vi "InitGantner.vi"(8 "error in":errorcluster, 10 "Port":i32) -> (0 "error out":errorcluster caption="error in", 2 "Module":T1)   [LabVIEW 2012]
uses:
  Gantner-Instruments ISMBUS32.llb/ISMBUS_Module.ctl
  Gantner-Instruments ISMBUS32.llb/ISMBUS_Channel.ctl
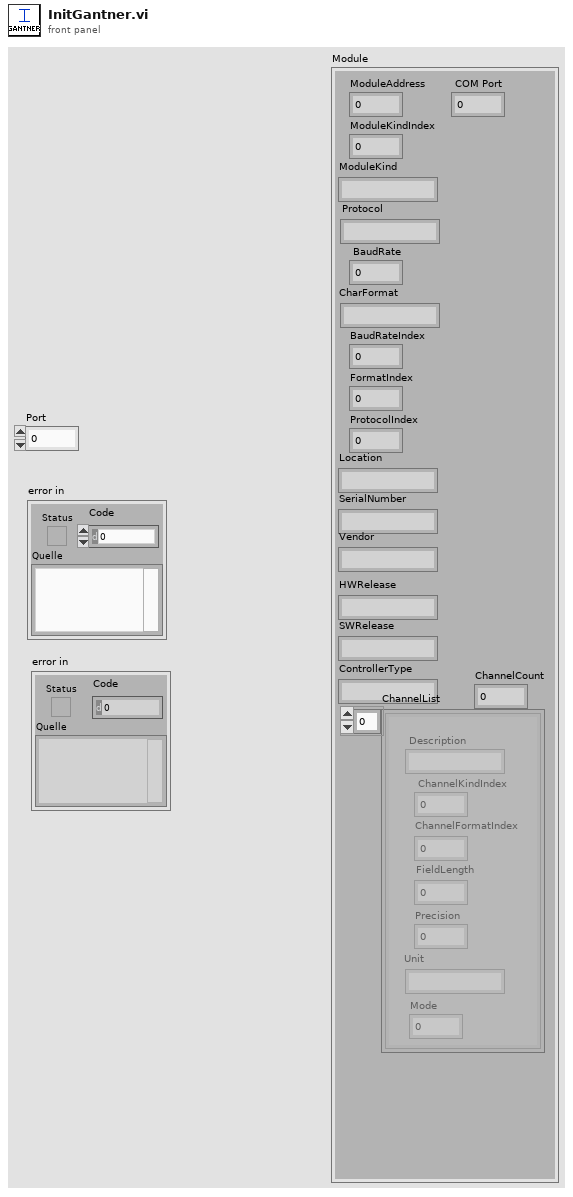
[diagram p1: front panel]
types:
  T1 = typedef "ISMBUS_Module.ctl" = cluster{"ModuleAddress":i32, "ModuleKindIndex":i32, "ModuleKind":string, " Protocol":string, " BaudRate":i32, "CharFormat":string, "BaudRateIndex":i32, "FormatIndex":i32, "ProtocolIndex":i32, "Location":string, "SerialNumber":string, "Vendor":string, "HWRelease":string, "SWRelease":string, "ControllerType":string, "ChannelList":T2[], "ChannelCount":i32, " COM Port":i32}
  T2 = typedef "ISMBUS_Channel.ctl" = cluster{" Description":string, " ChannelKindIndex":i32, "ChannelFormatIndex":i32, " FieldLength":i32, "Precision":i32, "Unit":string, "Mode":i32}
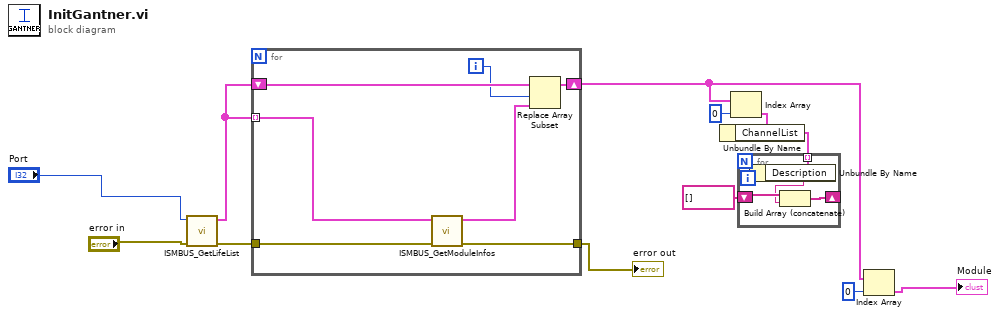
[diagram p0: block diagram]
diagram:
  n1 = call "ISMBUS_GetLifeList.vi"("Fehler (Eingang - kein Fehler)"="error in", "ComPort"="Port") -> ("Fehler (Ausgang)"=w11:errorcluster, "ModuleArray"=w10:T1[])  [unwired: 8 out]
  n2 = for {
    tunnel: w10 -> [w14] mode=indexing
    tunnel: w11 -> [w13]
    tunnel: [w16] -> w1
    shift-right: [w19] -> w8
    shift-left: w10 -> [w18]
    i -> [w17]
    n3 = call "ISMBUS_GetModuleInfos.vi"("Fehler (Eingang, kein Fehler)"=w13, "Module"=w14) -> ("Fehler (Ausgang)"=w16:errorcluster, "Module (Ausgang)"=w15:T1)  [unwired: 8 out]
    n4 = Replace Array Subset(array=w18, new element=w15, index=w17) -> (w19:T1[])
  }
  "error out" <- w1
  n5 = Index Array(array=w8, index=0 ("Index")) -> (element=w6:T1)
  n6 = Unbundle By Name(w6) -> ("ChannelList"=w5:T2[])
  n7 = for {
    tunnel: w5 -> [w23] mode=indexing
    shift-right: [w20] -> _
    shift-left: string[] [] -> [w22]
    n8 = Unbundle By Name(w23) -> ("Description"=w21:string)
    n9 = Build Array (concatenate)(w22, w21) -> (w20:string[])
  }
  n10 = Index Array(array=w8, index=0 ("Index")) -> (element=→"Module":T1)
